vi "ConfigUtilities - Add Channel.vi"(5 "Channel Path Sources":string[](array[string]), 6 "Rx Channel Name":string, 7 "Channel Path Destinations":string[](array[string]), 8 "error in (no error)":errorcluster, 9 "Rx Channel Ref":T1 format="%.0x", 10 "Dependent Node Ref":T1 format="%.0x", 11 "Rx Section Ref in":T1 format="%.0x") -> (0 "error out":errorcluster, 3 "Rx Section Ref in":T1 format="%.0x")   [LabVIEW 2016, in "UDP-Custom-Device System Explorer.lvlib"]
uses:
  UDP-Custom-Device System Explorer.lvlib
  <vilib>/NI Veristand/Custom Device API/Custom Device Item Ref.ctl
  <vilib>/NI Veristand/Custom Device API/Custom Device Channel.ctl
  <vilib>/NI Veristand/Custom Device API/Custom Device Channel Type.ctl
  Shared/Constants.vi
  <vilib>/NI Veristand/Custom Device API/Set Item Property (Dependent Node Pointer).vi
  <vilib>/NI VeriStand/Custom Device API/Custom Device API.lvlib
  Shared/UDP-Custom-Device Shared.lvlib
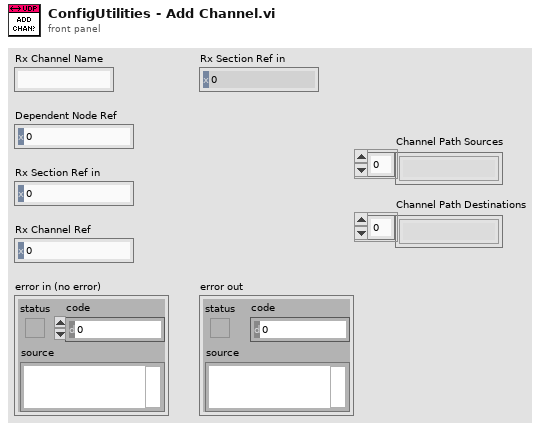
[diagram p1: front panel]
types:
  T1 = typedef "Custom Device API.lvlib/Custom Device Item Ref.ctl" = u64
  T2 = cluster{"Channel Names":string[], "Channel Paths":string[], "Dependent Node References":T1[]}
  T3 = typedef "Custom Device API.lvlib/Custom Device Channel.ctl" = cluster{"Type":T4, "Units":string, "Default Value":dbl, "Faultable":bool, "Scalable":bool}
  T4 = typedef "Custom Device API.lvlib/Custom Device Channel Type.ctl" = enum16{"Input", "Output"}
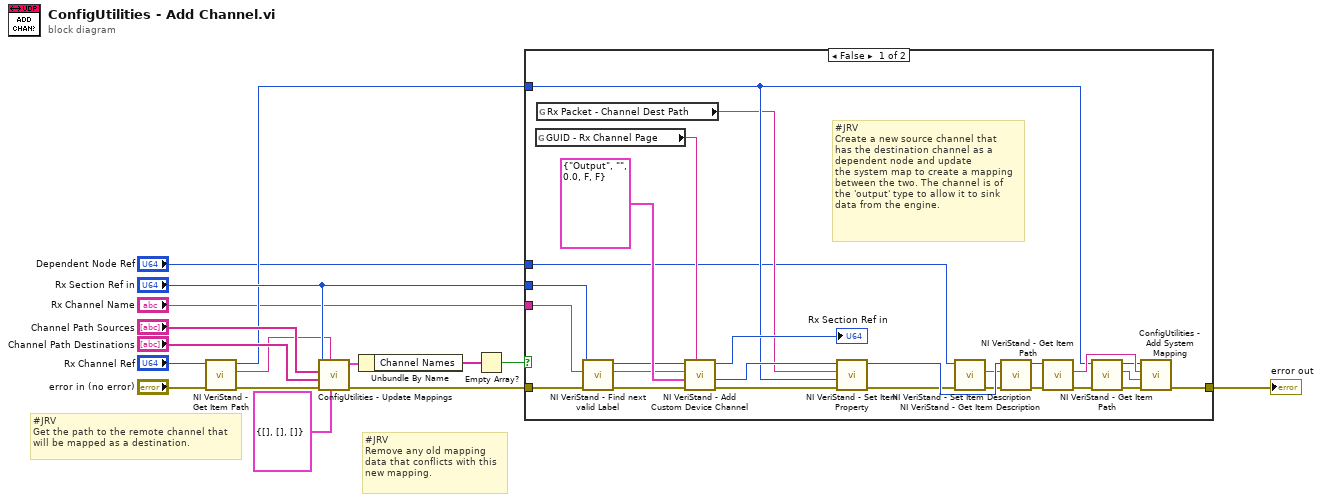
[diagram p0: block diagram]
diagram:
  # "#JRV\nRemove any old mapping\ndata that conflicts with this\nnew mapping."
  # "#JRV\nGet the path to the remote channel that\nwill be mapped as a destination."
  n1 = call <vilib>:"NI VeriStand - Get Item Path.vi"("error in (no error)"="error in (no error)", "Item Ref in"="Rx Channel Ref") -> ("error out"=w10:errorcluster, "Path"=w9:string, "Item Ref out"=w7:T1)  [unwired: 6 in, 1 out]
  n2 = call "ConfigUtilities - Update Mappings.vi"("Channel Data in"=T2 {"Channel Names"=[], "Channel Paths"=[], "Dependent Node References"=[]}, "Channel Path"=w9, "error in (no error)"=w10, "Channel Path Destinations"="Channel Path Destinations", "Channel Path Sources"="Channel Path Sources", "Item Ref in"="Rx Section Ref in") -> ("error out"=w4:errorcluster, "Channel Data out"=w6:T2)  [unwired: 4 in]
  n3 = Unbundle By Name(w6) -> ("Channel Names"=w5:string[])
  n4 = Empty Array?(array=w5) -> (empty?=w3:bool)
  n5 = case shown="False" w3 {
    tunnel: [w35 w43] -> w16
    tunnel: "Rx Section Ref in" -> [w23 _]
    tunnel: w7 -> [w22 _]
    tunnel: w4 -> [w21 w43]
    tunnel: "Dependent Node Ref" -> [w18 _]
    tunnel: "Rx Channel Name" -> [w17 _]
    frame False {
      # "#JRV\nCreate a new source channel that\nhas the destination channel as a \ndependent node and update\nthe system map to create a mapping\nbetween the two. The channel is of\nthe 'output' type to allow it to sink\ndata from the engine."
      n6 = global read "Constants.vi" "GUID - Rx Channel Page"() -> (w20:string)
      n7 = global read "Constants.vi" "Rx Packet - Channel Dest Path"() -> (w19:string)
      n8 = call <vilib>:"NI VeriStand - Find next valid Label.vi"("error in (no error)"=w21, "Label"=w17, "Item Ref in"=w23) -> ("error out"=w25:errorcluster, "Label out"=w26:string, "Item Ref out"=w24:T1)  [unwired: 4 in, 2 out]
      n9 = call <vilib>:"NI VeriStand - Add Custom Device Channel.vi"("GUID (Default Channel)"=w20, "error in (no error)"=w25, "Channel"=T3 {"Type"=enum."Output", "Units"="", "Default Value"=0.0, "Faultable"=FALSE, "Scalable"=FALSE}, "Channel Name"=w26, "Parent Ref in"=w24) -> ("error out"=w31:errorcluster, "Channel Ref"=w33:T1, "Parent Ref out"=→"Rx Section Ref in":T1)  [unwired: 3 in, 1 out]
      n10 = call-poly <vilib>:"NI VeriStand - Set Item Property.vi"("error in (no error)"=w31, "Dependent Node Ref"=w22, "Property Name"=w19, "Item Ref in"=w33) -> ("error out"=w32:errorcluster, "Item Ref out"=w34:T1)  [unwired: 5 in, 1 out]
      n11 = call <vilib>:"NI VeriStand - Get Item Description.vi"("error in (no error)"=w32, "Item Ref in"=w18) -> ("error out"=w28:errorcluster, "Description"=w29:string)  [unwired: 6 in, 2 out]
      n12 = call <vilib>:"NI VeriStand - Set Item Description.vi"("error in (no error)"=w28, "Description"=w29, "Item Ref in"=w34) -> ("error out"=w36:errorcluster, "Item Ref out"=w37:T1)  [unwired: 6 in, 1 out]
      n13 = call <vilib>:"NI VeriStand - Get Item Path.vi"("error in (no error)"=w36, "Item Ref in"=w37) -> ("error out"=w38:errorcluster, "Path"=w41:string)  [unwired: 6 in, 2 out]
      n14 = call <vilib>:"NI VeriStand - Get Item Path.vi"("error in (no error)"=w38, "Item Ref in"=w22) -> ("error out"=w39:errorcluster, "Path"=w42:string, "Item Ref out"=w40:T1)  [unwired: 6 in, 1 out]
      n15 = call "ConfigUtilities - Add System Mapping.vi"("error in (no error)"=w39, "Channel Path Destination"=w42, "Channel Path Source"=w41, "Item Ref in"=w40) -> ("error out"=w35:errorcluster)  [unwired: 6 in, 1 out]
    }
    frame True {
    }
  }
  "error out" <- w16
